vi "Sort group metadata.vi"(0 "reference in":refnum<class "metadata.lvclass">, 5 "error in (no error)":errorcluster) -> (14 "reference out":refnum<class "metadata.lvclass">, 19 "error out":errorcluster)   [LabVIEW 2019, in "metadata.lvclass"]
uses:
  metadata.lvclass
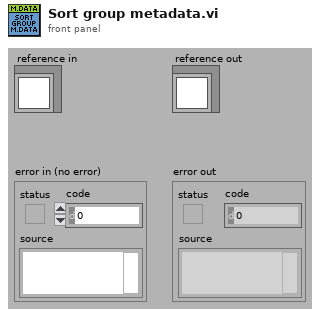
[diagram p1: front panel]
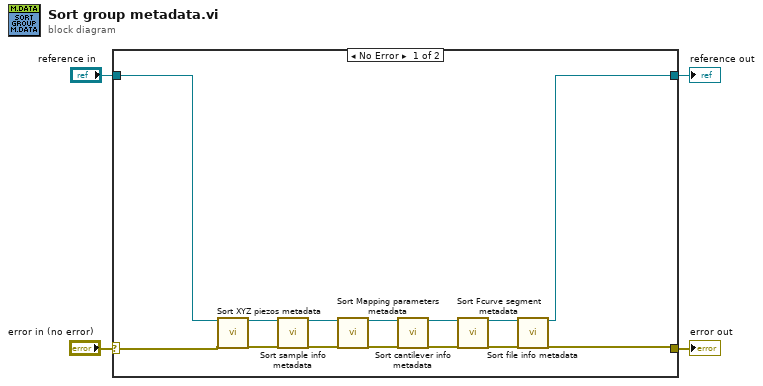
[diagram p0: block diagram]
diagram:
  n1 = case shown="No Error" "error in (no error)" {
    selector: "error in (no error)" -> [w11 w20]
    tunnel: [w5 w20] -> w3
    tunnel: [w12 w19] -> w1
    tunnel: "reference in" -> [w13 w19]
    frame No Error {
      n2 = call "Sort XYZ piezos metadata.vi"("reference in"=w13, "error in (no error)"=w11) -> ("reference out"=w18:refnum<class "metadata.lvclass">, "error out"=w10:errorcluster)  [unwired: 15 in, 1 out]
      n3 = call "Sort sample info metadata.vi"("reference in"=w18, "error in (no error)"=w10) -> ("reference out"=w17:refnum<class "metadata.lvclass">, "error out"=w9:errorcluster)  [unwired: 15 in, 1 out]
      n4 = call "Sort Mapping parameters metadata.vi"("reference in"=w17, "error in (no error)"=w9) -> ("reference out"=w16:refnum<class "metadata.lvclass">, "error out"=w8:errorcluster)  [unwired: 15 in, 1 out]
      n5 = call "Sort cantilever info metadata.vi"("reference in"=w16, "error in (no error)"=w8) -> ("reference out"=w15:refnum<class "metadata.lvclass">, "error out"=w7:errorcluster)  [unwired: 15 in, 1 out]
      n6 = call "Sort Fcurve segment metadata.vi"("reference in"=w15, "error in (no error)"=w7) -> ("reference out"=w14:refnum<class "metadata.lvclass">, "error out"=w6:errorcluster)  [unwired: 16 in]
      n7 = call "Sort file info metadata.vi"("reference in"=w14, "error in (no error)"=w6) -> ("reference out"=w12:refnum<class "metadata.lvclass">, "error out"=w5:errorcluster)  [unwired: 15 in, 1 out]
    }
    frame Error {
    }
  }
  "error out" <- w3
  "reference out" <- w1
